vi "静态调用串口基本配置对话框.vi"() -> ()   [LabVIEW 2013]
uses:
  <vilib>/Platform/TimedLoop/XDataNode/timing_clust.ctl
  <vilib>/Platform/TimedLoop/XDataNode/nitl_modes.ctl
  <vilib>/Platform/TimedLoop/XDataNode/wakeup.ctl
  <vilib>/Platform/TimedLoop/XDataNode/XDataNode.xnode
  <vilib>/Platform/TimedLoop/XDataNode/XDNodeRunTimeDep.lvlib
panel:
  out "应用程序:所有内存中的VI":string[](array[string])
  in  "串口基本配置对话框":bool
  in  "停止":bool
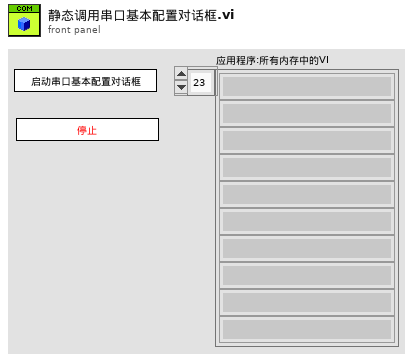
[diagram p1: front panel]
types:
  T1 = typedef "XDNodeRunTimeDep.lvlib/timing_clust.ctl" = cluster{"Expected End [f-1]":u64, "Actual End [f-1]":u64, "Finished Late? [f-1]":bool, "Expected End [i-1]":u64, "Actual End [i-1]":u64, "Finished Late? [i-1]":bool, "Expected Start [i]":u64, "Actual Start [i]":u64, "Expected Start [f]":u64, "Actual Start [f]":u64, "Source Name":string, "Structure Name":string, "Period":i64, "Deadline":i64, "Offset":i64, "Start":i64, "Priority":i32, "Timeout":i32, "Mode":T2, "Wakeup Reason":T3, "Error":errorcluster, "Source Type":string, "Secondary Source Type":string, "Global End Time":u64, "Global Start Time":u64, "Frame Duration":u64, "Iteration Duration":u64, "Assigned CPU":i32, "I/O Scan Engine Mode":u32}
  T2 = typedef "XDNodeRunTimeDep.lvlib/nitl_modes.ctl" = enum32{"No Change", "Process missed periods, maintain original phase", "Discard missed periods, maintain original phase", "Process missed periods, ignore original phase", "Discard missed periods, ignore original phase"}
  T3 = typedef "XDNodeRunTimeDep.lvlib/wakeup.ctl" = enum32{"Normal", "Aborted", "Asynchronous wakeup", "Timing source error", "Timed loop error", "Timeout"}
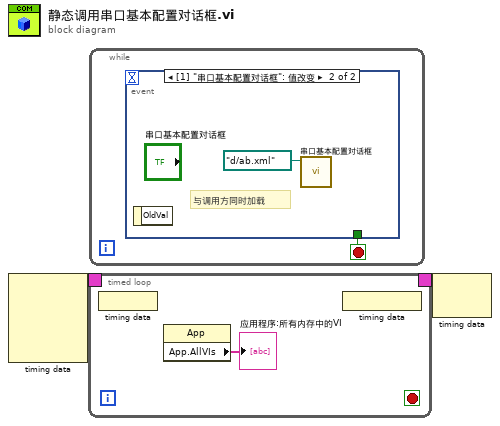
[diagram p0: block diagram]
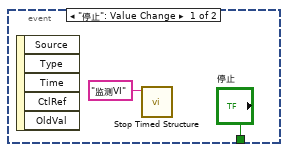
[diagram p2: hidden frame]
diagram:
  n1 = node-c288() -> (w2:T1)  [unwired: 4 in]
  n2 = timed-loop {
    timing: w2 -> [_]
    timing-out: [_] -> w1
    stop <- _ stop-if-true
    n3 = node-c288() -> ()  [unwired: 1 in]
    n4 = property class="App"() -> ("App.AllVIs"=→"应用程序:所有内存中的VI":string[])  [unwired: 2 in, 2 out]
    n5 = node-c288() -> ()  [unwired: 1 out]
  }
  n6 = while {
    stop <- w6 stop-if-true
    n7 = event shown="[1] \"串口基本配置对话框\": 值改变" {
      selector: _ -> [_ _]
      dyn-events: _ -> [_ _]
      timeout: _ -> [_ _]
      tunnel: ["停止" _] -> w6
      event "停止": Value Change {
        n8 = event-data() -> ()  [unwired: 1 in, 5 out]
        n9 = call <vilib>:"Stop Timed Structure.vi"("name"="监测VI") -> ()  [unwired: 10 in, 1 out]
      }
      event "串口基本配置对话框": Value Change {
        # "与调用方同时加载"
        n10 = event-data() -> ()  [unwired: 1 in, 1 out]
        n11 = call "串口基本配置对话框.vi"("XML File Path"=path "d:/ab.xml") -> ()  [unwired: 11 in]
      }
    }
  }
  n12 = node-c288(w1) -> ()  [unwired: 1 out]
